vi "GPIO Read.vi"(9 "pPinValue":u32, 10 "PinMask":u32, 11 "DevHandle":i32) -> (1 "pPinValue out":u32, 3 "function return":i32)   [LabVIEW 2010, in "usb2gpio.lvlib"]
doc: "int WINAPI GPIO_Read(int DevHandle,unsigned int PinMask, unsigned int *pPinValue);"
uses:
  usb2gpio.lvlib
  USB2XXX.dll
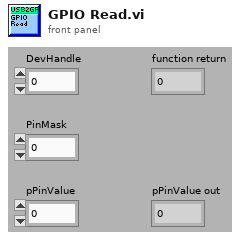
[diagram p1: front panel]
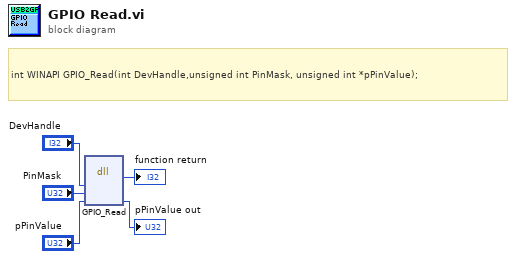
[diagram p0: block diagram]
diagram:
  # "int WINAPI GPIO_Read(int DevHandle,unsigned int PinMask, unsigned int *pPinValue);"
  n1 = dll-call lib="G:/OtherWork/USB2XXX_Example/trunk/Labview/PublicFiles/usb2gpio/USB2XXX.*" fn="GPIO_Read"("DevHandle"="DevHandle", "PinMask"="PinMask", "pPinValue"="pPinValue") -> (→"function return":i32, "pPinValue"=→"pPinValue out":u32)  [unwired: 5 in, 2 out]
